vi "Format LV Error as JSON Data.vi"(10 "error in":errorcluster) -> (0 "error out":errorcluster, 2 "Error Value out":variant)   [LabVIEW 2020, in "JSON-RPC Lib.lvlib" / "JSONRPC Server.lvclass"]
doc: "This converts a LabVIEW Error to a JSON Tree for use with \"Add Response - Server Error\"."
uses:
  JSONRPC Server.lvclass
  Variant Data Manipulation/Insert Element at Start.vi
  Variant Data Manipulation/Variant Data Manipulation.lvlib
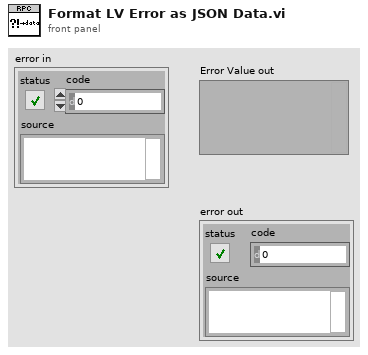
[diagram p1: front panel]
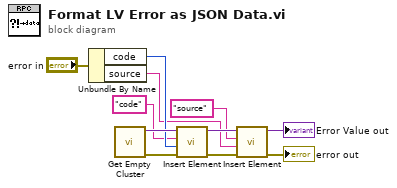
[diagram p0: block diagram]
diagram:
  n1 = Unbundle By Name("error in") -> ("code"=w4:i32, "source"=w1:string)
  n2 = call "Get Empty Cluster.vi"() -> ("error out"=w5:errorcluster, "Variant (Cluster) out"=w10:variant)  [unwired: 10 in]
  n3 = call-poly "Insert Element.vi"("error in (no error)"=w5, "element"=w4, "Name"="code", "Variant (Cluster) in"=w10) -> ("error out"=w6:errorcluster, "Variant (Cluster) out"=w9:variant)  [unwired: 6 in]
  n4 = call-poly "Insert Element.vi"("error in (no error)"=w6, "element"=w1, "Name"="source", "Variant (Cluster) in"=w9) -> ("error out"=→"error out":errorcluster, "Variant (Cluster) out"=→"Error Value out":variant)  [unwired: 6 in]
